vi "MakeExample.vi"(8 "error in (no error)":errorcluster, 9 "TriggerRefractoryPeriod (Frames)":i32, 10 "StimulusObject Parameters":variant, 11 "JustTailEllipseRatioRails in":refnum<class "JustTailEllipseRatioRails.lvclass">) -> (0 "error out":errorcluster, 3 "JustTailEllipseRatioRails out":refnum<class "JustTailEllipseRatioRails.lvclass">)   [LabVIEW 2019, in "JustTailEllipseRatioRails.lvclass"]
uses:
  JustTailEllipseRatioRails.lvclass
  JustTailEllipseRatioRailsInputCluster.ctl
  JustTailEllipseRatioRails.lvclass/JustTailEllipseRatioRails.ctl
  ParametersGlobal.vi
  StimulusObject.lvclass
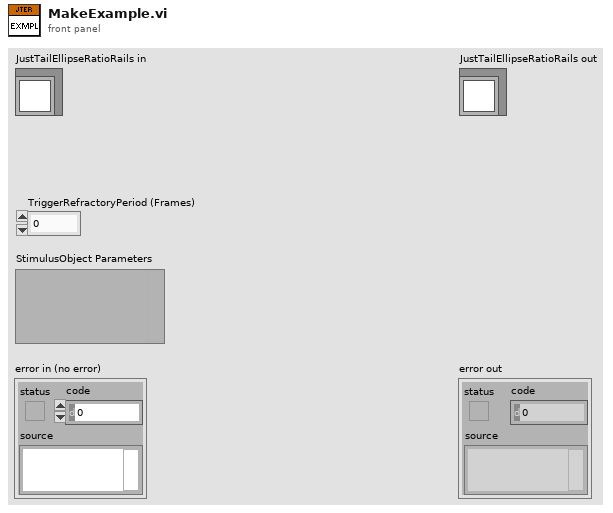
[diagram p1: front panel]
types:
  T1 = typedef "JustTailEllipseRatioRails.lvclass/JustTailEllipseRatioRailsInputCluster.ctl" = cluster{"Constant Intensity (uW/mm^2, negative is blue)":sgl, "dot radius (mm)":sgl, "Intensities (uW/mm^2, negative is blue)":sgl[], "Durations (s)":sgl[], "Inter trigger interval (s)":dbl, "Ellipse Ratio Trigger Point":sgl}
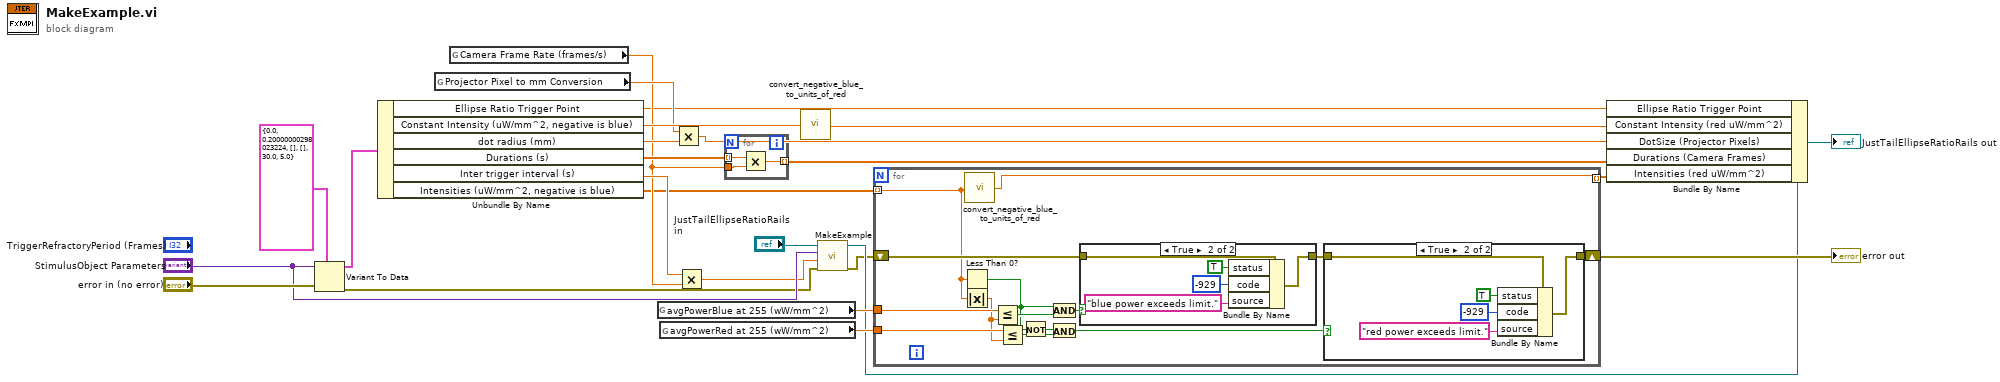
[diagram p0: block diagram]
diagram:
  n1 = Variant To Data(error in="error in (no error)", type=T1 {"Constant Intensity (uW/mm^2, negative is blue)"=0.0, "dot radius (mm)"=0.2, "Intensities (uW/mm^2, negative is blue)"=[], "Durations (s)"=[], "Inter trigger interval (s)"=30.0, "Ellipse Ratio Trigger Point"=5.0} ("JustTailEllipseRatioRailsInputCluster"), Variant="StimulusObject Parameters") -> (data=w25:T1, error out=w4:errorcluster)
  n2 = Unbundle By Name(w25) -> ("Ellipse Ratio Trigger Point"=w11:sgl, "Constant Intensity (uW/mm^2, negative is blue)"=w23:sgl, "dot radius (mm)"=w21:sgl, "Durations (s)"=w18:sgl[], "Inter trigger interval (s)"=w24:dbl, "Intensities (uW/mm^2, negative is blue)"=w15:sgl[])
  n3 = global read "ParametersGlobal.vi" "Projector Pixel to mm Conversion"() -> (w20:sgl)
  n4 = global read "ParametersGlobal.vi" "Camera Frame Rate (frames/s)"() -> (w17:sgl)
  n5 = global read "ParametersGlobal.vi" "avgPowerBlue at 255 (wW/mm^2)"() -> (w14:sgl)
  n6 = global read "ParametersGlobal.vi" "avgPowerRed at 255 (wW/mm^2)"() -> (w13:sgl)
  n7 = Multiply(x=w20, y=w21) -> (x*y=w19:sgl)
  n8 = Multiply(x=w24, y=w17) -> (x*y=w5:dbl)
  n9 = for {
    tunnel: w18 -> [w28] mode=indexing
    tunnel: w17 -> [w27]
    tunnel: [w26] -> w16 mode=indexing
    n10 = Multiply(x=w28, y=w27) -> (x*y=w26:sgl)
  }
  n11 = call "convert_negative_blue_to_units_of_red.vi"("Intensity in units of red (positive) and blue (negative)"=w23) -> ("Intensity in units of red (positive and negative)"=w22:sgl)
  n12 = call-parent "MakeExample.vi"("error in (no error)"=w4, "TriggerRefractoryPeriod (Frames)"=w5, "StimulusObject Parameters"="StimulusObject Parameters", "StimulusObject in"="JustTailEllipseRatioRails in") -> ("error out"=w2:errorcluster, "StimulusObject out"=w3:refnum<class "JustTailEllipseRatioRails.lvclass">)  [unwired: 6 in]
  n13 = for {
    tunnel: w15 -> [w36] mode=indexing
    shift-right: [w40] -> w8
    shift-left: w2 -> [w41]
    tunnel: w14 -> [w39]
    tunnel: w13 -> [w38]
    tunnel: [w37] -> w12 mode=indexing
    n14 = Less Than 0?(x=w36) -> (x < 0?=w29:bool)
    n15 = Absolute Value(x=w36) -> (abs(x)=w35:sgl)
    n16 = call "convert_negative_blue_to_units_of_red.vi"("Intensity in units of red (positive) and blue (negative)"=w36) -> ("Intensity in units of red (positive and negative)"=w37:sgl)
    n17 = Less Or Equal?(x=w39, y=w35) -> (x <= y?=w34:bool)
    n18 = Less Or Equal?(x=w38, y=w35) -> (x <= y?=w31:bool)
    n19 = Not(x=w29) -> (.not. x?=w30:bool)
    n20 = And(x=w29, y=w34) -> (x .and. y?=w33:bool)
    n21 = And(x=w30, y=w31) -> (x .and. y?=w32:bool)
    n22 = case shown="True" w33 {
      tunnel: w41 -> [w49 w54]
      tunnel: [w49 w53] -> w42
      frame False {
      }
      frame True {
        n23 = Bundle By Name(cluster=w54, "status"=TRUE, "code"=-929, "source"="blue power exceeds limit.") -> (w53:errorcluster)
      }
    }
    n24 = case shown="True" w32 {
      tunnel: w42 -> [w43 w48]
      tunnel: [w43 w47] -> w40
      frame False {
      }
      frame True {
        n25 = Bundle By Name(cluster=w48, "status"=TRUE, "code"=-929, "source"="red power exceeds limit.") -> (w47:errorcluster)
      }
    }
  }
  "error out" <- w8
  n26 = Bundle By Name(cluster=w3, "Ellipse Ratio Trigger Point"=w11, "Constant Intensity (red uW/mm^2)"=w22, "DotSize (Projector Pixels)"=w19, "Durations (Camera Frames)"=w16, "Intensities (red uW/mm^2)"=w12) -> (→"JustTailEllipseRatioRails out":refnum<class "JustTailEllipseRatioRails.lvclass">)
